vi "Fetch.vi"(8 "error in (no error)":errorcluster, 10 "Message in":refnum<class "FetchMessage.lvclass">, 11 "Example Class B in":refnum<class "ExampleClassB.lvclass">) -> (0 "error out":errorcluster, 3 "Example Class B out":refnum<class "ExampleClassB.lvclass">)   [LabVIEW 2012, in "ExampleClassB.lvclass"]
doc: "Fetches data received from observee via a \"fetch\" message. Displays the data on the main.vi front panel via a indicator reference."
uses:
  ExampleClassB.lvclass
  <vilib>/Distrio/Murmex/FetchMessage/FetchMessage.lvclass
  <vilib>/Distrio/Murmex/Murmex/Murmex.lvclass
  ExampleClassB.lvclass/ExampleClassB.ctl
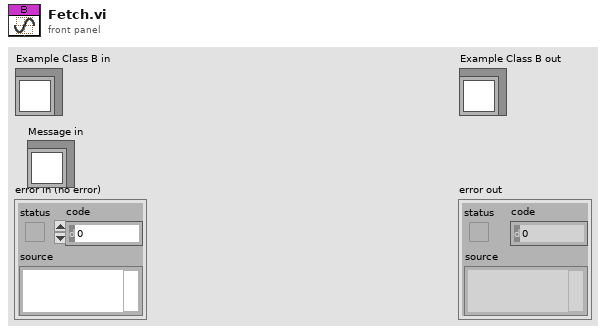
[diagram p1: front panel]
types:
  T1 = typedef "Murmex.lvlib/FetchMessage.lvclass/Channel data cluster.ctl" = cluster{"channel id":i32, "data UInt8":u8[], "data type":T2, "dimensions":i32[], "physical units":T3[], "waveform dt":dbl, "waveform":T4}
  T2 = typedef "Murmex.lvlib/Murmex.lvclass/data_type_enum.ctl" = enum16{"Float128", "Float64", "Float32", "Int64", "Int32", "Int16", "Int8", "UInt64", "UInt32", "UInt16", "UInt8", "Boolean", "String"}
  T3 = typedef "Murmex.lvlib/Murmex.lvclass/Physical Units.ctl" = cluster{"Base Units":enum16{"radian", "steradian", "second", "meter", "kilogram", "ampere", "kelvin", "mole", "candela"}, "Exponent":i16}
  T4 = typedef "Murmex.lvlib/Murmex.lvclass/waveform_type_enum.ctl" = enum16{"no waveform", "analog", "digital"}
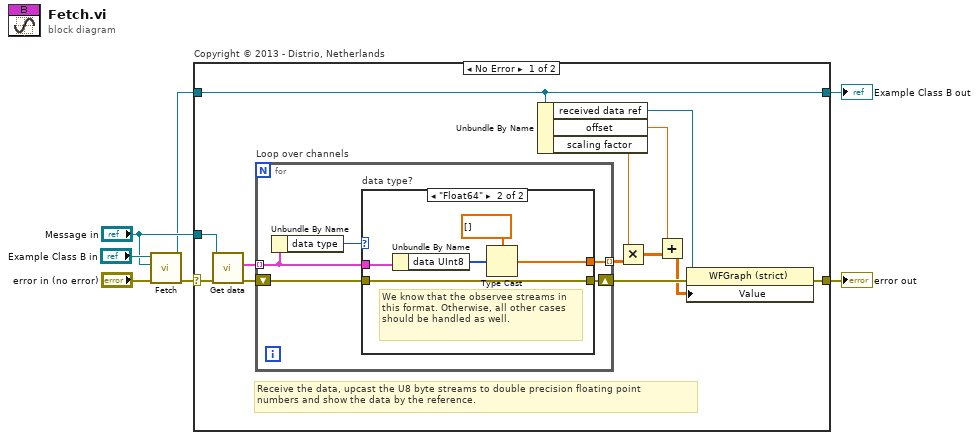
[diagram p0: block diagram]
diagram:
  n1 = call-parent "Fetch.vi"("error in (no error)"="error in (no error)", "Message in"="Message in", "Murmex in"="Example Class B in") -> ("error out"=w5:errorcluster, "Murmex out"=w1:refnum<class "ExampleClassB.lvclass">)  [unwired: 7 in]
  n2 = case "Copyright © 2013 - Distrio, Netherlands" shown="No Error" w5 {
    selector: w5 -> [w18 w32]
    tunnel: [w14 w33] -> w4
    tunnel: w1 -> [w14 w33]
    tunnel: [w15 w32] -> w3
    tunnel: "Message in" -> [w20 _]
    frame No Error {
      # "Receive the data, upcast the U8 byte streams to double precision floating point\nnumbers and show the data by the reference."
      n3 = call <vilib>:"Get data.vi"("error in (no error)"=w18, "FetchMessage.lvclass"=w20) -> ("error out"=w19:errorcluster, "data (channels)"=w8:T1[])  [unwired: 7 in, 1 out]
      n4 = for "Loop over channels" {
        tunnel: [w23] -> w12 mode=indexing
        tunnel: w8 -> [w22] mode=indexing
        shift-right: [w24] -> w16
        shift-left: w19 -> [w25]
        n5 = Unbundle By Name(w22) -> ("data type"=w21:T2)
        n6 = case "data type?" shown="\"Float64\"" w21 {
          tunnel: w22 -> [_ w28]
          tunnel: [w26 w31] -> w24
          tunnel: w25 -> [w26 w31]
          tunnel: [_ w30] -> w23
          frame Default {
          }
          frame "Float64" {
            # "We know that the observee streams in this format. Otherwise, all other cases should be handled as well."
            n7 = Unbundle By Name(w28) -> ("data UInt8"=w27:u8[])
            n8 = Type Cast(type=dbl[] [] ("data (UInt8)"), x=w27) -> (*(type *) &x=w30:dbl[])
          }
        }
      }
      n9 = Unbundle By Name(w14) -> ("received data ref"=w17:refnum<vi>, "offset"=w9:dbl, "scaling factor"=w13:dbl)
      n10 = Multiply(x=w13, y=w12) -> (x*y=w11:dbl[][])
      n11 = Add(x=w9, y=w11) -> (x+y=w10:dbl[][])
      n12 = property class="WFGraph (strict)"(reference=w17, error in=w16, "Value"=w10) -> (error out=w15:errorcluster)  [unwired: 1 out]
    }
    frame Error {
    }
  }
  "error out" <- w3
  "Example Class B out" <- w4
